vi "SerialReadString.vi"(8 "error in (no error)":errorcluster, 11 "VISA Refnum in":refnum<visa-resource-name>) -> (0 "error out":errorcluster, 2 "trimmed string":string, 3 "VISA Refnum out":refnum<visa-resource-name>)   [LabVIEW 2014]
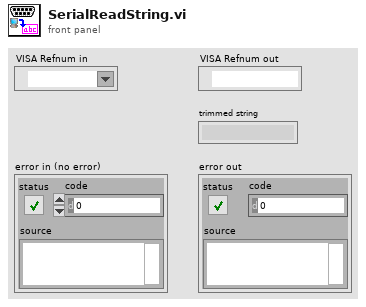
[diagram p1: front panel]
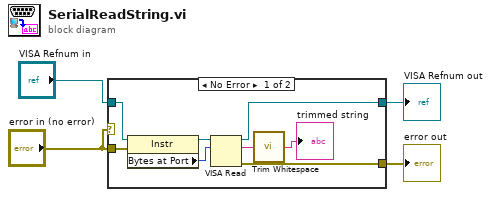
[diagram p0: block diagram]
diagram:
  n1 = case shown="No Error" "error in (no error)" {
    tunnel: "error in (no error)" -> [w9 w13]
    tunnel: "VISA Refnum in" -> [w8 w14]
    tunnel: [w7 w13] -> w3
    tunnel: [w6 w14] -> w2
    frame No Error {
      n2 = property class="Instr"(reference=w8, error in=w9) -> (reference out=w5:refnum<visa-resource-name>, "Bytes at Port"=w10:u32)  [unwired: 1 out]
      n3 = VISA Read(VISA resource name=w5, byte count=w10) -> (VISA resource name out=w6:refnum<visa-resource-name>, read buffer=w11:string, error out=w7:errorcluster)  [unwired: 1 in, 1 out]
      n4 = call <vilib>:"Trim Whitespace.vi"("string"=w11) -> ("trimmed string"=→"trimmed string":string)  [unwired: 1 in]
    }
    frame Error {
    }
  }
  "error out" <- w3
  "VISA Refnum out" <- w2
